vi "Read Voltage Datas.vi"   [LabVIEW 2023, in "vmmsolib.lvlib"]
doc: "DLL_API unsigned int WINAPI ReadVoltageDatas(char channel, double* buffer, unsigned int length);"
uses:
  vmmsolib.lvlib
  vmmso.dll
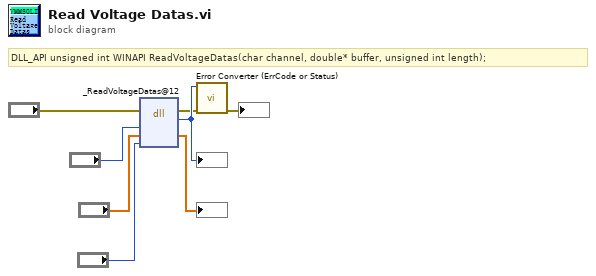
[diagram p0: block diagram]
diagram:
  # "DLL_API unsigned int WINAPI ReadVoltageDatas(char channel, double* buffer, unsigned int length);"
  n1 = dll-call lib="D:/VmMsoSDK/demo-Labview/2023/vmmsolib/vmmso.*" fn="_ReadVoltageDatas@12"(error in="?", "channel"="?", "buffer"="?", "length"="?") -> (error out=w2:errorcluster, w8:u32, "buffer"=→"?":dbl[])  [unwired: 4 in, 1 out]
  "?" <- w8
  n2 = call "Error Converter (ErrCode or Status).vi"("error in (no error)"=w2, "error code"=w8) -> ("error out"=→"?":errorcluster)  [unwired: 9 in]
